vi "USS9804_GetDevInfo.vi"(8 "Error In":errorcluster, 11 "Handle":u64) -> (0 "Error Out":errorcluster, 1 "devADbit":i32, 2 "devFifoSize":i32, 3 "Handle 2":u64, 5 "devVer":i32)   [LabVIEW 2015]
uses:
  USS9804.DLL
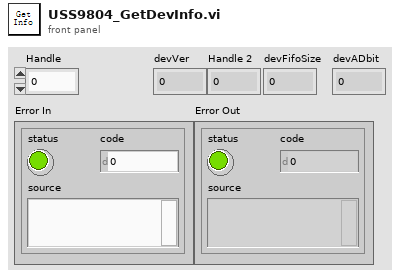
[diagram p1: front panel]
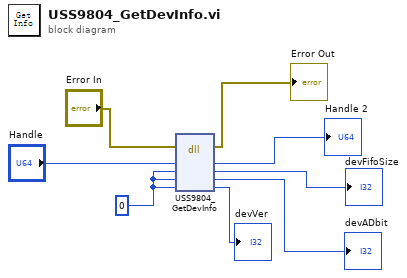
[diagram p0: block diagram]
diagram:
  w5 = 0 ("devFifoSize")
  n1 = dll-call lib="PTH2Sabs CYexinrongWorkplace\t普密斯Thickness-measurementLabVIEWUSS9804.DLL" fn="USS9804_GetDevInfo"(error in="Error In", "Handle"="Handle", "devFifoSize"=w5, "devADbit"=w5, "devVer"=w5) -> (error out=→"Error Out":errorcluster, "Handle"=→"Handle 2":u64, "devFifoSize"=→"devFifoSize":i32, "devADbit"=→"devADbit":i32, "devVer"=→"devVer":i32)  [unwired: 3 in, 1 out]
